vi "Stop Acq.vi"(8 "error in (no error)":errorcluster, 11 "Image Acquisition in":refnum<class "Image Acquisition.lvclass">) -> (0 "error out":errorcluster, 3 "Image Acquisition out":refnum<class "Image Acquisition.lvclass">)   [LabVIEW 2016, in "Image Acquisition.lvlib" / "Image Acquisition.lvclass"]
uses:
  Image Acquisition.lvclass
  Image Acquisition.lvclass/Image Acquisition.ctl
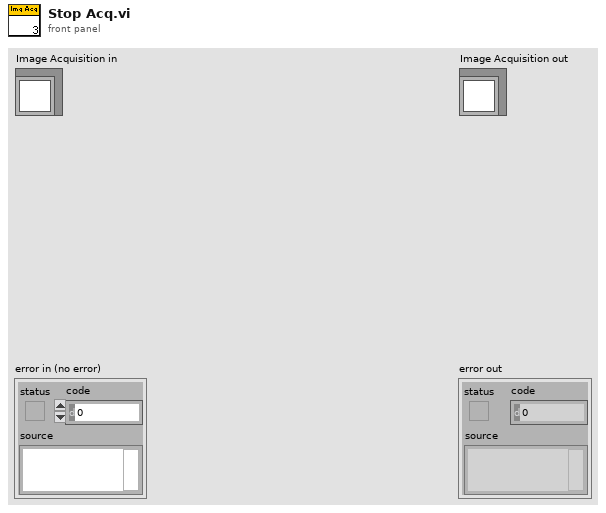
[diagram p1: front panel]
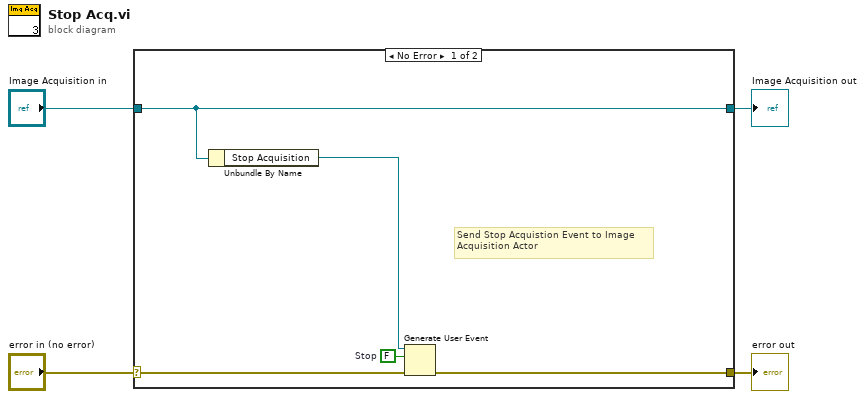
[diagram p0: block diagram]
diagram:
  n1 = case shown="No Error" "error in (no error)" {
    selector: "error in (no error)" -> [w8 w11]
    tunnel: [w7 w11] -> w3
    tunnel: [w9 w10] -> w1
    tunnel: "Image Acquisition in" -> [w9 w10]
    frame No Error {
      w5 = FALSE  # Stop
      # "Send Stop Acquistion Event to Image\nAcquisition Actor"
      n2 = Unbundle By Name(w9) -> ("Stop Acquisition"=w6:refnum<user-event>)
      n3 = Generate User Event(user event=w6, event data cluster=w5, error in=w8) -> (error out=w7:errorcluster)  [unwired: 1 in, 1 out]
    }
    frame Error {
    }
  }
  "error out" <- w3
  "Image Acquisition out" <- w1
